vi "Close VISA Resource.vi"(8 "error in (no error)":errorcluster, 11 "Connection Info in":T1={"VISA Resource"="", "Address"=1} {"Address" min=1}) -> (0 "error out":errorcluster)   [LabVIEW 2020, in "plugin_flodx_pressure.lvlib" / "plugin.lvlib" / "Instrument Manager.lvlib"]
doc: "Close the VISA resource connection. Calls mock drivers if symbol NO_DRIVER == 1."
uses:
  Instrument Manager.lvlib
  connection_info/Connection Info.ctl
  mock_driver/mock_driver.lvlib
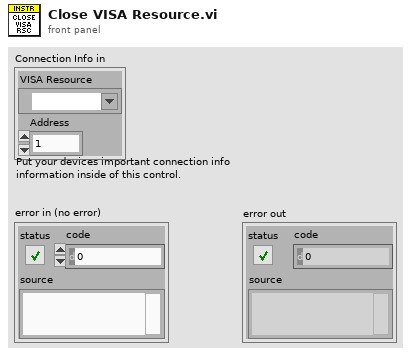
[diagram p1: front panel]
types:
  T1 = typedef "plugin_flodx_pressure.lvlib/plugin.lvlib/Instrument Manager.lvlib/Connection Info.ctl" = cluster{"VISA Resource":refnum<visa-resource-name>, "Address":u8}
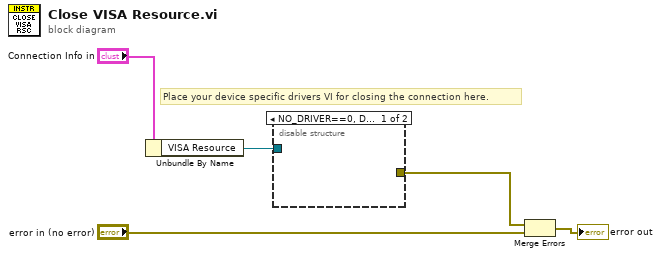
[diagram p0: block diagram]
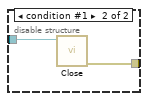
[diagram p2: hidden frame]
diagram:
  # "Place your device specific drivers VI for closing the connection here."
  n1 = Unbundle By Name("Connection Info in") -> ("VISA Resource"=w1:refnum<visa-resource-name>)
  n2 = disable-structure shown="NO_DRIVER==0, Default" {
    disable-tunnel: [_ w7] -> w5
    disable-tunnel: w1 -> [_ w6]
    frame condition #0 (active) {
    }
    frame condition #1 {
      n3 = call "Close.vi"("VISA resource name"=w6) -> ("Error out"=w7:errorcluster)  [unwired: 10 in]
    }
  }
  n4 = Merge Errors(w5, "error in (no error)") -> (→"error out":errorcluster)
